vi "IED watchdogReset.vi"(8 "error in":errorcluster, 11 "SCADA in":refnum<class "EMS.lvclass">) -> (0 "error out":errorcluster, 3 "SCADA out":refnum<class "EMS.lvclass">)   [LabVIEW 2018, in "EMS Core.lvlib" / "EMS.lvclass"]
uses:
  EMS.lvclass
  C:/Users/Administrator/Desktop/LabVIEW EMS/EMS Generic Actor/EMS Generic/EMS Generic.lvclass
  <vilib>/ORNL/CSEISMIC DDS/CSEISMIC DDS Base/Data Types/Controls/Timestamp.ctl
  EMS Generic Actor/EMS Generic/EMS Generic.lvclass/EMS Generic.ctl
  EMS.lvclass/EMS.ctl
  <vilib>/ORNL/CSEISMIC DDS/CSEISMIC DDS Base/Data Types/IED_Status.ctl
  <vilib>/ORNL/CSEISMIC DDS/CSEISMIC DDS Base/Data Types/Controls/DeviceID.ctl
  <vilib>/ActorFramework/Message Enqueuer/Message Enqueuer.lvclass/Message Enqueuer.ctl
  <vilib>/ActorFramework/Message Enqueuer/Enqueue.vi
  IED Actors/IED Actor/IED Messages/Watchdog Reset Msg/Watchdog Reset Msg.lvclass
  C:/Program Files (x86)/National Instruments/LabVIEW 2018/vi.lib/ActorFramework/Message/Message.lvclass
  <vilib>/ActorFramework/Message Priority Queue/Priority Enqueue.vi
  <vilib>/ORNL/CSEISMIC DDS/CSEISMIC DDS Base/CSEISMIC DDS.lvclass
  EMS Generic Actor/EMS Generic/EMS Generic.lvclass
  Utilities/Status Messaging.llb/Status Messaging.lvlib
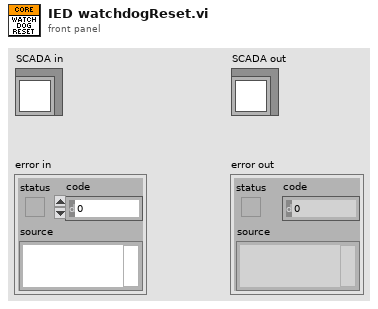
[diagram p1: front panel]
types:
  T1 = typedef "CSEISMIC DDS.lvlib/CSEISMIC DDS.lvclass/Timestamp.ctl" = cluster{"Seconds":u64, "Remainder":u64}
  T2 = typedef "CSEISMIC DDS.lvlib/CSEISMIC DDS.lvclass/IED_Status.ctl" = cluster{"DeviceID":T3, "Timestamp":T1, "MicrogridID":u8, "Active":bool, "Inactive":bool, "Error":i32, "Fault":bool, "ErrorString":string}
  T3 = typedef "CSEISMIC DDS.lvlib/CSEISMIC DDS.lvclass/DeviceID.ctl" = string
  T4 = typedef "EMS Generic Actor.lvlib/EMS Generic.lvclass/Data Type DVRs.ctl" = cluster{"IED_Status":refnum<data-value>, "IED_Status_0":refnum<data-value>, "DER_Measurement":refnum<data-value>, "DER_Info":refnum<data-value>, "DER_Status":refnum<data-value>, "ES_Measurement":refnum<data-value>, "ES_Info":refnum<data-value>, "PV_Info":refnum<data-value>, "SmartRelay_Info":refnum<data-value>, "SmartRelay_Measurement":refnum<data-value>, "Meter_Info":refnum<data-value>, "Meter_Measurement":refnum<data-value>, "HVAC_Status":refnum<data-value>, "HVAC_Measurement":refnum<data-value>, "PriceData_RealTime":refnum<data-value>, "PriceData_Demand":refnum<data-value>, "PriceData_Energy":refnum<data-value>, "ForecastData_Long":refnum<data-value>, "ForecastData_Short":refnum<data-value>, "DER_Control":refnum<data-value>, "DER_SetPointF":refnum<data-value>, "DER_SetPointP":refnum<data-value>, "DER_SetPointQ":refnum<data-value>, "DER_SetPointPF":refnum<data-value>, "DER_SetPointV":refnum<data-value>, "PV_setCurtailment":refnum<data-value>, "PV_setRampRate":refnum<data-value>, "Relay_Control":refnum<data-value>, "Load_Control":refnum<data-value>, "HVAC_Control":refnum<data-value>, "Generator_Info":refnum<data-value>, "ForecastData_Long_Backup":refnum<data-value>, "PriceData_RealTime_Backup":refnum<data-value>}
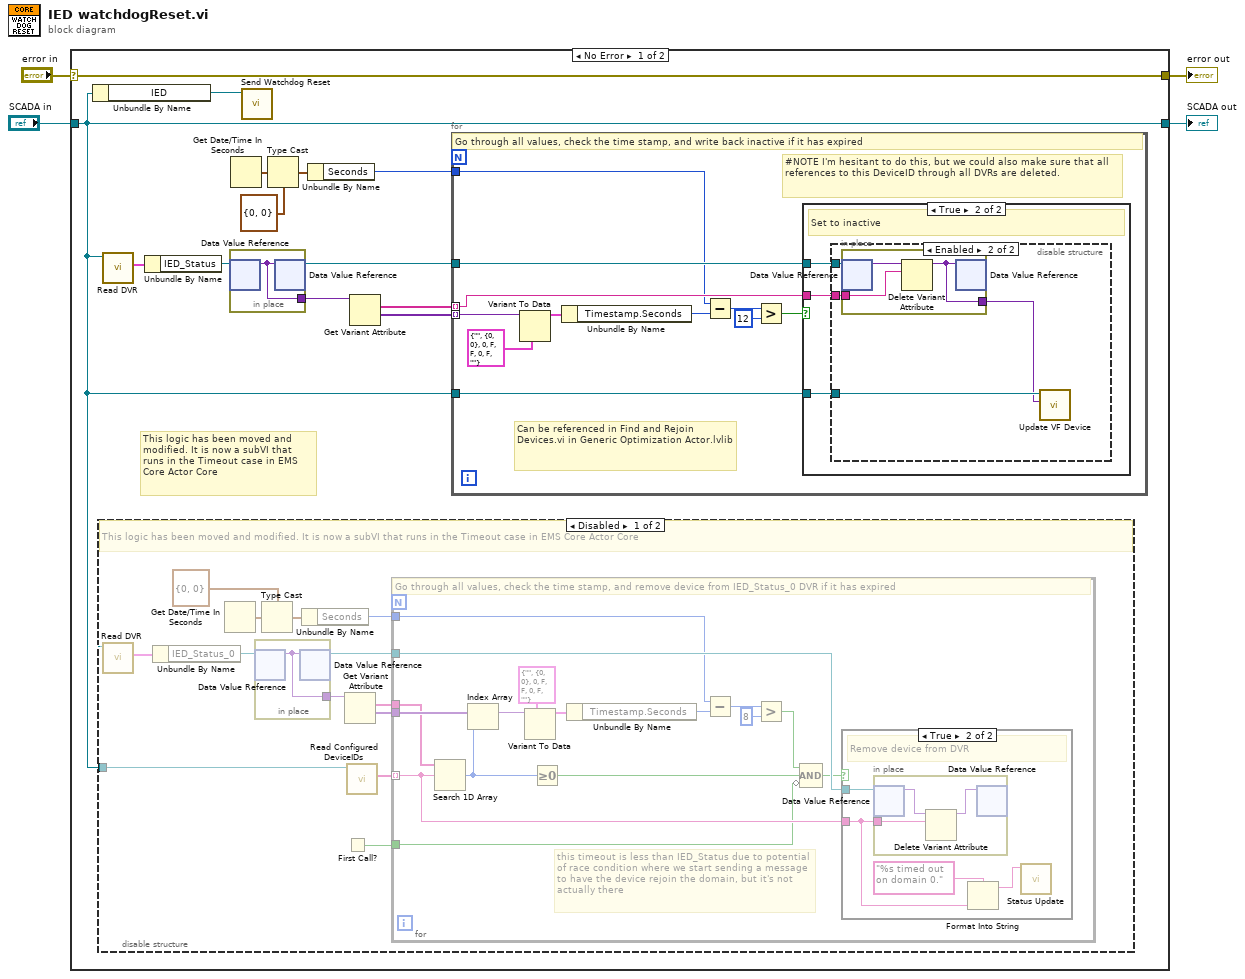
[diagram p0: block diagram]
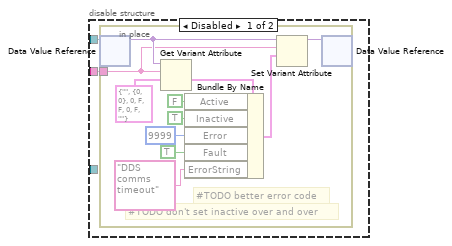
[diagram p5: hidden frame]
diagram:
  n1 = case shown="No Error" "error in" {
    selector: "error in" -> [w17 w91]
    tunnel: [w17 w91] -> w3
    tunnel: [w5 w90] -> w1
    tunnel: "SCADA in" -> [w5 w90]
    frame No Error {
      # "This logic has been moved and modified. It is now a subVI that runs in the Timeout case in EMS Core Actor Core"
      n2 = Unbundle By Name(w5) -> ("IED"=w16:refnum<class "Message Enqueuer.lvclass">)
      n3 = disable-structure shown="Disabled" {
        disable-tunnel: w5 -> [w19 _]
        frame Disabled {
          # "This logic has been moved and modified. It is now a subVI that runs in the Timeout case in EMS Core Actor Core"
          n4 = call "Read DVR.vi"("EMS Generic in"=w19) -> ("DVR"=w18:T4)  [unwired: 9 in, 1 out]
          n5 = Unbundle By Name(w18) -> ("IED_Status_0"=w30:refnum<data-value>)
          n6 = Get Date/Time In Seconds() -> (seconds since 1Jan1904=w23:timestamp)
          n7 = in-place {
            in-place-border: [w31] -> w28
            n8 = in-place-dvr #1(w30) -> (w31:variant)  [unwired: 1 out]
            n9 = in-place-dvr #1(w31) -> (w29:refnum<data-value>)  [unwired: 1 out]
          }
          n10 = Type Cast(type=T1 {"Seconds"=0, "Remainder"=0} ("Timestamp"), x=w23) -> (*(type *) &x=w25:T1)
          n11 = Unbundle By Name(w25) -> ("Seconds"=w22:u64)
          n12 = First Call?() -> (First Call?: T/F=w20:bool)
          n13 = Get Variant Attribute(Variant=w28) -> (names=w27:string[], values=w26:variant[])  [unwired: 3 in, 2 out]
          n14 = call "Read Configured DeviceIDs.vi"("EMS Generic in"=w19) -> ("DeviceIDs"=w21:T3[])  [unwired: 8 in, 2 out]
          n15 = for {
            tunnel: w26 -> [w47]
            tunnel: w27 -> [w36]
            tunnel: w29 -> [w42]
            tunnel: w22 -> [w40]
            tunnel: w21 -> [w33] mode=indexing
            tunnel: w20 -> [w32]
            # "this timeout is less than IED_Status due to potential of race condition where we start sending a message to have the device rejoin the domain, but it's not actually there"
            # "Go through all values, check the time stamp, and remove device from IED_Status_0 DVR if it has expired"
            n16 = Search 1D Array(1D array=w36, element=w33) -> (index of element=w34:i32)  [unwired: 1 in]
            n17 = Index Array(array=w47, index=w34) -> (element=w35:variant)
            n18 = Variant To Data(type=T2 {"DeviceID"="", "Timestamp"={"Seconds"=0, "Remainder"=0}, "MicrogridID"=0, "Active"=FALSE, "Inactive"=FALSE, "Error"=0, "Fault"=FALSE, "ErrorString"=""} ("IED_Status"), Variant=w35) -> (data=w46:T2)  [unwired: 1 in, 1 out]
            n19 = Greater Or Equal To 0?(x=w34) -> (x >= 0?=w38:bool)
            n20 = Unbundle By Name(w46) -> ("Timestamp.Seconds"=w45:u64)
            n21 = Subtract(x=w40, y=w45) -> (x-y=w44:u64)
            n22 = Greater?(x=w44, y=u64 8) -> (0:w39:bool)
            n23 = Compound Arithmetic op=AND(w39, w38, invert w32) -> (w37:bool)
            n24 = case shown="True" w37 {
              tunnel: w42 -> [_ w51]
              tunnel: w33 -> [_ w49]
              frame False {
                # "Do nothing"
              }
              frame True {
                # "Remove device from DVR"
                n25 = in-place {
                  in-place-border: w49 -> [w53]
                  n26 = in-place-dvr #2(w51) -> (w54:variant)  [unwired: 1 out]
                  n27 = Delete Variant Attribute(6:w53, 7:w54) -> (3:w52:variant)  [unwired: 1 in, 2 out]
                  n28 = in-place-dvr #2(w52) -> ()  [unwired: 2 out]
                }
                n29 = Format Into String(format string="%s timed out on domain 0.", w49) -> (resulting string=w48:string)  [unwired: 2 in, 1 out]
                n30 = call "Status Update.vi"("Status Update"=w48) -> ()  [unwired: 9 in, 2 out]
              }
            }
          }
        }
        frame Enabled {
        }
      }
      n31 = call "Read DVR.vi"("EMS Generic in"=w5) -> ("DVR"=w6:T4)  [unwired: 9 in, 1 out]
      n32 = Unbundle By Name(w6) -> ("IED_Status"=w15:refnum<data-value>)
      n33 = in-place {
        in-place-border: [w55] -> w14
        n34 = in-place-dvr #3(w15) -> (w55:variant)  [unwired: 1 out]
        n35 = in-place-dvr #3(w55) -> (w11:refnum<data-value>)  [unwired: 1 out]
      }
      n36 = Get Date/Time In Seconds() -> (seconds since 1Jan1904=w8:timestamp)
      n37 = call "Send Watchdog Reset.vi"("Message Enqueuer"=w16) -> ()  [unwired: 9 in, 2 out]
      n38 = Type Cast(type=T1 {"Seconds"=0, "Remainder"=0} ("Timestamp"), x=w8) -> (*(type *) &x=w10:T1)
      n39 = Unbundle By Name(w10) -> ("Seconds"=w7:u64)
      n40 = Get Variant Attribute(Variant=w14) -> (names=w12:string[], values=w13:variant[])  [unwired: 3 in, 2 out]
      n41 = for {
        tunnel: w13 -> [w66] mode=indexing
        tunnel: w12 -> [w59] mode=indexing
        tunnel: w11 -> [w60]
        tunnel: w7 -> [w57]
        tunnel: w5 -> [w56]
        # "Can be referenced in Find and Rejoin Devices.vi in Generic Optimization Actor.lvlib"
        # "#NOTE I'm hesitant to do this, but we could also make sure that all references to this DeviceID through all DVRs are deleted."
        # "Go through all values, check the time stamp, and write back inactive if it has expired"
        n42 = Variant To Data(type=T2 {"DeviceID"="", "Timestamp"={"Seconds"=0, "Remainder"=0}, "MicrogridID"=0, "Active"=FALSE, "Inactive"=FALSE, "Error"=0, "Fault"=FALSE, "ErrorString"=""} ("IED_Status"), Variant=w66) -> (data=w65:T2)  [unwired: 1 in, 1 out]
        n43 = Unbundle By Name(w65) -> ("Timestamp.Seconds"=w64:u64)
        n44 = Subtract(x=w57, y=w64) -> (x-y=w63:u64)
        n45 = Greater?(x=w63, y=u64 12) -> (0:w61:bool)
        n46 = case shown="True" w61 {
          tunnel: w60 -> [_ w69]
          tunnel: w59 -> [_ w68]
          tunnel: w56 -> [_ w67]
          frame False {
            # "Do nothing"
          }
          frame True {
            # "Set to inactive"
            n47 = disable-structure shown="Enabled" {
              disable-tunnel: w69 -> [w71 w86]
              disable-tunnel: w68 -> [w70 w85]
              disable-tunnel: w67 -> [_ w84]
              frame Disabled {
                n48 = in-place {
                  in-place-border: w70 -> [w77]
                  # "#TODO don't set inactive over and over"
                  # "#TODO better error code"
                  n49 = in-place-dvr #4(w71) -> (w79:variant)  [unwired: 1 out]
                  n50 = Get Variant Attribute(Variant=w79, name=w77, default value (empty Variant)=T2 {"DeviceID"="", "Timestamp"={"Seconds"=0, "Remainder"=0}, "MicrogridID"=0, "Active"=FALSE, "Inactive"=FALSE, "Error"=0, "Fault"=FALSE, "ErrorString"=""} ("IED_Status")) -> (value=w82:T2)  [unwired: 1 in, 3 out]
                  n51 = Bundle By Name(cluster=w82, "Active"=FALSE, "Inactive"=TRUE, "Error"=9999, "Fault"=TRUE, "ErrorString"="DDS comms timeout") -> (w76:T2)
                  n52 = Set Variant Attribute(Variant=w79, name=w77, value=w76) -> (Variant out=w78:variant)  [unwired: 1 in, 2 out]
                  n53 = in-place-dvr #4(w78) -> ()  [unwired: 2 out]
                }
              }
              frame Enabled {
                n54 = in-place {
                  in-place-border: w85 -> [w88]
                  in-place-border: [w87] -> w83
                  n55 = in-place-dvr #5(w86) -> (w89:variant)  [unwired: 1 out]
                  n56 = Delete Variant Attribute(6:w88, 7:w89) -> (3:w87:variant)  [unwired: 1 in, 2 out]
                  n57 = in-place-dvr #5(w87) -> ()  [unwired: 2 out]
                }
                n58 = call "Update VF Device.vi"("IED_Status"=w83, "EMS in"=w84) -> ()  [unwired: 10 in]
              }
            }
          }
        }
      }
    }
    frame Error {
    }
  }
  "error out" <- w3
  "SCADA out" <- w1
